vi "fake_image_pixel_count.vi"(1 "pixel counter":u16) -> (0 "input cluster":T1)   [LabVIEW 2010]
uses:
  common_typedefs/channels_cluster.ctl
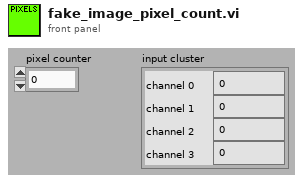
[diagram p1: front panel]
types:
  T1 = typedef "channels_cluster.ctl" = cluster{"channel 0":u32, "channel 1":u32, "channel 2":u32, "channel 3":u32}
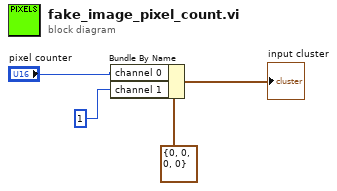
[diagram p0: block diagram]
diagram:
  n1 = Bundle By Name(cluster=T1 {"channel 0"=0, "channel 1"=0, "channel 2"=0, "channel 3"=0} ("input cluster"), "channel 0"="pixel counter", "channel 1"=u16 1 ("f")) -> (→"input cluster":T1)
